vi "Horizontal Concatinate Image Data.vi"   [LabVIEW 2020, in "image.lvlib"]
doc: "Horizontally Concatinate Image Data Arrays."
uses:
  image.lvlib
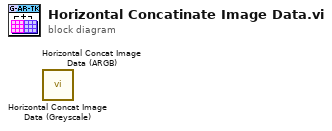
[diagram p0: block diagram]
diagram:
  n1 = call "Horizontal Concat Image Data (Greyscale).vi"() -> ()  [unwired: 2 in, 1 out]
  n2 = call "Horizontal Concat Image Data (ARGB).vi"() -> ()  [unwired: 2 in, 1 out]
